vi "PXI-4130 Channel Section Page.vi"(8 "error in (no error)":errorcluster, 11 "Node Ptr":T3 format="%.0x") -> (0 "error out":errorcluster)   [LabVIEW 2009, in "PXI-4130 Custom Device.lvlib"]
uses:
  PXI-4130 Custom Device.lvlib
  <vilib>/NI VeriStand/Custom Device API/Custom Device Item Ref.ctl
  Channel Sense.ctl
  Channel Type.ctl
  <vilib>/NI VeriStand/Custom Device API/Get Item Property (I32).vi
  PXI-4130 Global Variable.vi
  <vilib>/NI VeriStand/Custom Device API/Set Item Property (I32).vi
  <vilib>/NI VeriStand/Custom Device API/Custom Device API.lvlib
panel:
  in  "Apply Change":bool
  in  "Channel Type":T1 caption="Channel 0 Sense" items=["Voltage Controlled", "Current Controlled"]
  in  "Channel Sense":T2=1008 caption="Channel 0 Sense" items=["Local"=1008, "Remote"=1009]
  in  "Header":cluster{"Section Name":string}={"Section Name"="Custom Device Item Settings"}
  in  "Description":string
  in  "Name":string
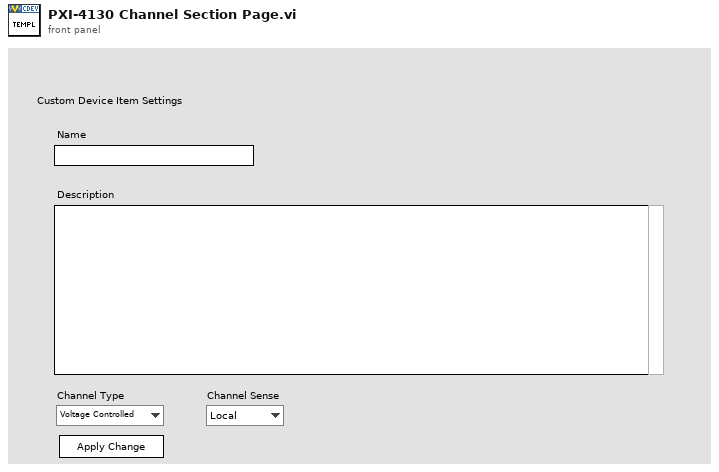
[diagram p1: front panel]
types:
  T1 = typedef "PXI-4130 Custom Device.lvlib/Channel Type.ctl" = i32
  T2 = typedef "PXI-4130 Custom Device.lvlib/Channel Sense.ctl" = i32
  T3 = typedef "Custom Device API.lvlib/Custom Device Item Ref.ctl" = u64
  T4 = enum8{"Enabled", "Disabled", "Disabled and Grayed Out"}
  T5 = typedef "Custom Device API.lvlib/Custom Device Item Info.ctl" = cluster{"Name":string, "Is Channel":bool, "GUID":string}
  T6 = typedef "Custom Device API.lvlib/Custom Device Commands.ctl" = enum16{"Default", "Item renamed", "Shutdown"}
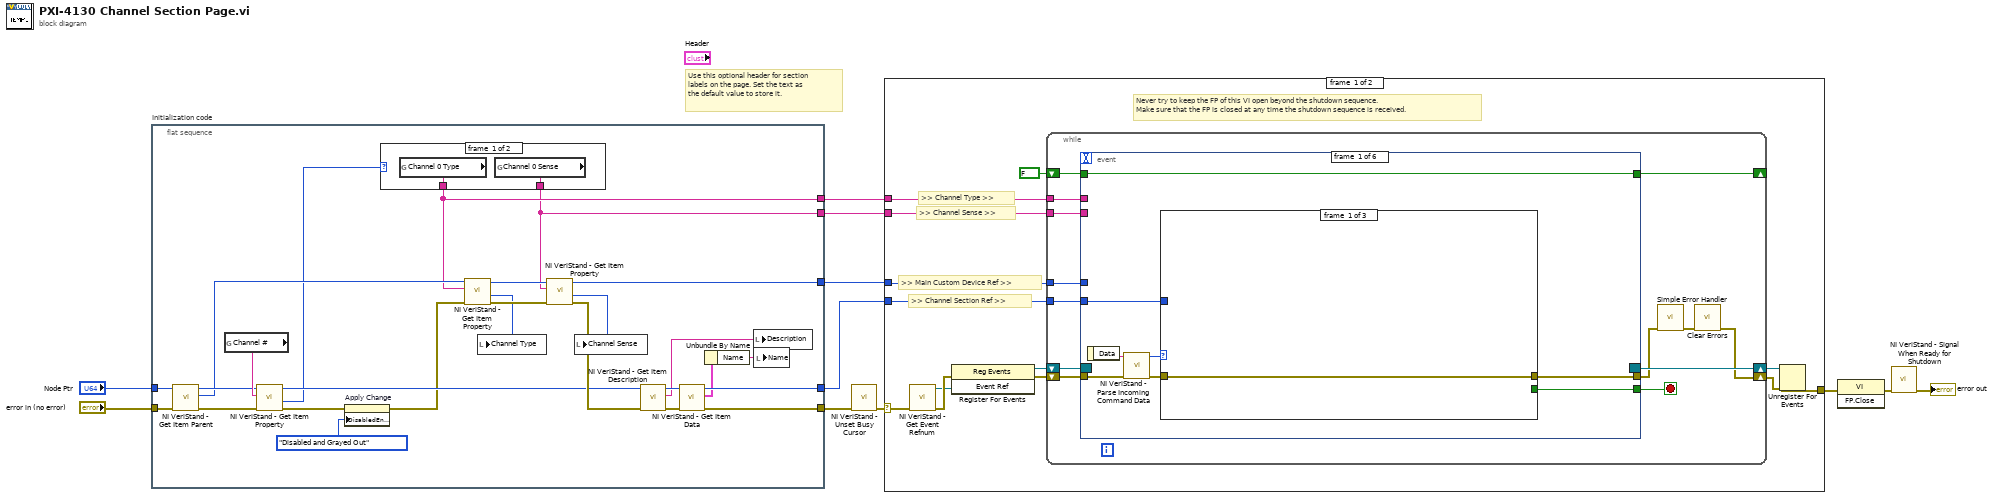
[diagram p0: block diagram]
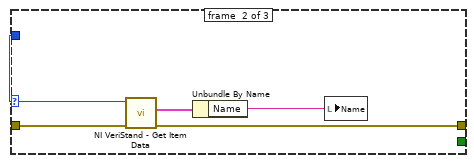
[diagram p2: hidden frame]
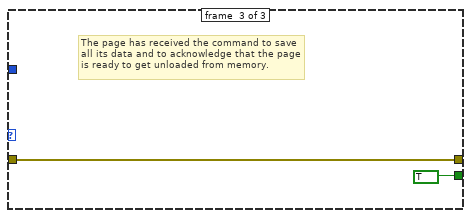
[diagram p3: hidden frame]
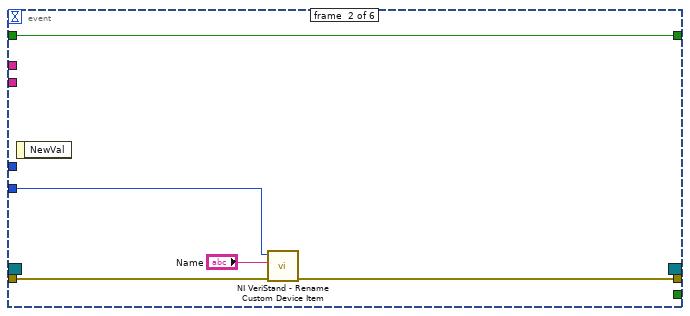
[diagram p4: hidden frame]
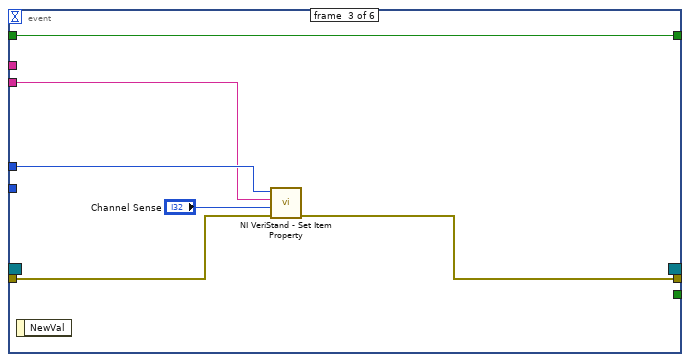
[diagram p5: hidden frame]
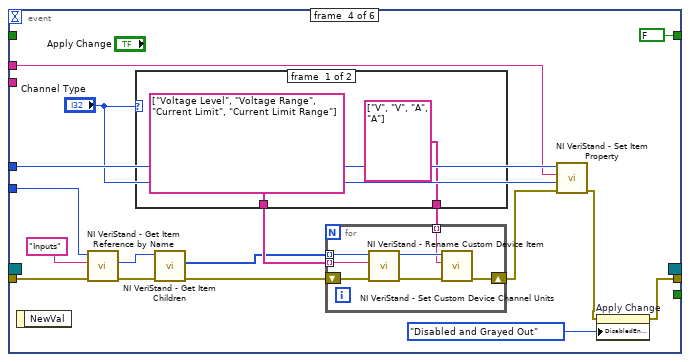
[diagram p6: hidden frame]
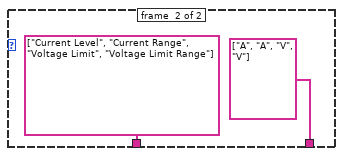
[diagram p7: hidden frame]
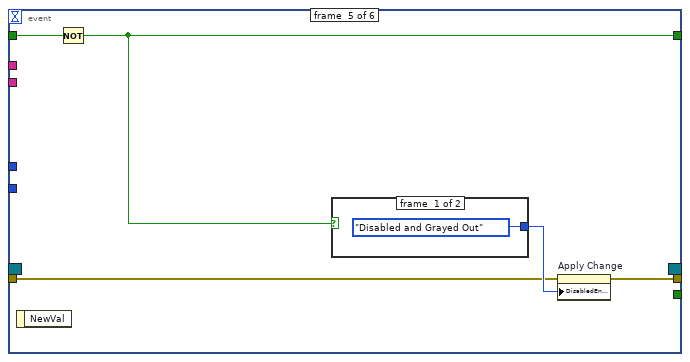
[diagram p8: hidden frame]
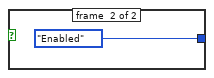
[diagram p9: hidden frame]
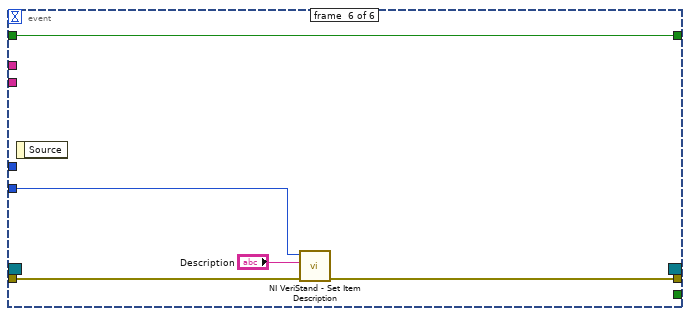
[diagram p10: hidden frame]
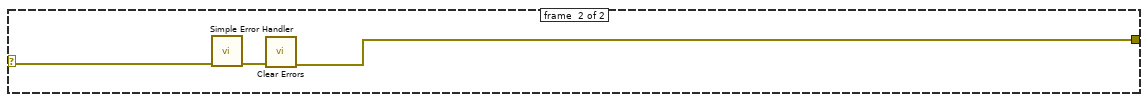
[diagram p11: hidden frame]
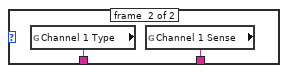
[diagram p12: hidden frame]
diagram:
  # "Use this optional header for section labels on the page. Set the text as the default value to store it."
  n1 = flat-sequence "Initialization code" {
    tunnel: "error in (no error)" -> [w28]
    tunnel: "Node Ptr" -> [w29]
    tunnel: [w31] -> w7
    tunnel: [w37] -> w4
    tunnel: [w18] -> w3
    tunnel: [w12] -> w2
    tunnel: [w13] -> w1
    frame #0 {
      n2 = call <vilib>:"NI VeriStand - Get Item Parent.vi"("error in (no error)"=w28, "Parent Ref in"=w29) -> ("error out"=w26:errorcluster, "Parent Ref"=w19:T3, "Parent Ref out"=w27:T3)  [unwired: 6 in, 1 out]
      n3 = global read "PXI-4130 Global Variable.vi" "Channel #"() -> (w30:string)
      n4 = call-poly <vilib>:"NI VeriStand - Get Item Property.vi"("error in (no error)"=w26, "Property Name"=w30, "Item Ref in"=w27) -> ("error out"=w16:errorcluster, "Value"=w14:i32, "Item Ref out"=w20:T3)  [unwired: 5 in, 1 out]
      n5 = property on="Apply Change" class="Bool"(error in=w16, "DisabledEnum"=T4."Disabled and Grayed Out" ("Disabled")) -> (error out=w15:errorcluster)  [unwired: 1 in, 1 out]
      n6 = case shown="0, Default" w14 {
        tunnel: [w39 w41] -> w13
        tunnel: [w38 w40] -> w12
        frame #0 {
          n7 = global read "PXI-4130 Global Variable.vi" "Channel 0 Type"() -> (w39:string)
          n8 = global read "PXI-4130 Global Variable.vi" "Channel 0 Sense"() -> (w38:string)
        }
        frame #1 {
          n9 = global read "PXI-4130 Global Variable.vi" "Channel 1 Type"() -> (w41:string)
          n10 = global read "PXI-4130 Global Variable.vi" "Channel 1 Sense"() -> (w40:string)
        }
      }
      n11 = call-poly <vilib>:"NI VeriStand - Get Item Property.vi"("error in (no error)"=w15, "Property Name"=w13, "Item Ref in"=w19) -> ("error out"=w24:errorcluster, "Value"=w22:i32, "Item Ref out"=w25:T3)  [unwired: 5 in, 1 out]
      n12 = local write "Channel Type"(w22) -> ()
      n13 = call-poly <vilib>:"NI VeriStand - Get Item Property.vi"("error in (no error)"=w24, "Property Name"=w12, "Item Ref in"=w25) -> ("error out"=w23:errorcluster, "Value"=w21:i32, "Item Ref out"=w18:T3)  [unwired: 5 in, 1 out]
      n14 = local write "Channel Sense"(w21) -> ()
      n15 = call <vilib>:"NI VeriStand - Get Item Description.vi"("error in (no error)"=w23, "Item Ref in"=w20) -> ("error out"=w34:errorcluster, "Description"=w35:string, "Item Ref out"=w36:T3)  [unwired: 7 out]
      n16 = call <vilib>:"NI VeriStand - Get Item Data.vi"("error in (no error)"=w34, "Item Ref in"=w36) -> ("error out"=w31:errorcluster, "Item Info"=w33:T5, "Item Ref out"=w37:T3)  [unwired: 7 out]
      n17 = Unbundle By Name(w33) -> ("Name"=w32:string)
      n18 = local write "Description"(w35) -> ()
      n19 = local write "Name"(w32) -> ()
    }
  }
  n20 = call <vilib>:"NI VeriStand - Unset Busy Cursor.vi"("error in (no error)"=w7) -> ("error out"=w6:errorcluster)  [unwired: 10 out]
  n21 = case shown="No Error" w6 {
    selector: w6 -> [w46 w137]
    tunnel: [w51 w135] -> w11
    tunnel: w4 -> [w47 _]
    tunnel: w3 -> [w45 _]
    tunnel: w2 -> [w44 _]
    tunnel: w1 -> [w43 _]
    frame #0 {
      # ">> Channel Type >>"
      # ">> Channel Sense >>"
      # ">> Main Custom Device Ref >>"
      # ">> Channel Section Ref >>"
      # "Never try to keep the FP of this VI open beyond the shutdown sequence.\nMake sure that the FP is closed at any time the shutdown sequence is received."
      n22 = call <vilib>:"NI VeriStand - Get Event Refnum.vi"("error in (no error)"=w46) -> ("error out"=w54:errorcluster, "Event Ref"=w50:refnum<user-event>)  [unwired: 9 out]
      n23 = register-events(error in=w54, w50) -> (reference out=w48:refnum<event-registration>, error out=w49:errorcluster)  [unwired: 1 in]
      n24 = while {
        tunnel: w47 -> [w63]
        shift-right: [w60] -> w52
        shift-left: w49 -> [w66]
        shift-right: [w67] -> w53
        shift-left: w48 -> [w65]
        tunnel: w45 -> [w59]
        tunnel: w44 -> [w58]
        tunnel: w43 -> [w57]
        shift-right: [w55] -> _
        shift-left: FALSE -> [w56]
        stop <- w64 stop-if-true
        n25 = event shown="[3] \"Apply Change\": Value Change" {
          selector: w65 -> [_ _ _ _ _ _]
          dyn-events: [_ _ _ _ _ _] -> w67
          timeout: _ -> [_ _ _ _ _ _]
          tunnel: w66 -> [w75 w88 w94 w108 w126 w133]
          tunnel: [w71 _ _ _ _ _] -> w64
          tunnel: [w70 w87 w93 w96 w125 w132] -> w62
          tunnel: w63 -> [w69 w86 _ w111 _ w134]
          tunnel: w59 -> [_ _ w91 w102 _ _]
          tunnel: w58 -> [_ _ w90 _ _ _]
          tunnel: w57 -> [_ _ _ w101 _ _]
          tunnel: w56 -> [w68 w84 w89 _ w124 w130]
          tunnel: [w68 w84 w89 FALSE w123 w130] -> w55
          event #0 {
            n26 = event-data() -> ("Data"=w74:string)  [unwired: 1 out]
            n27 = call <vilib>:"NI VeriStand - Parse Incoming Command Data.vi"("error in (no error)"=w75, "Data"=w74) -> ("error out"=w73:errorcluster, "Action"=w72:T6)  [unwired: 8 out]
            n28 = case shown="\"Shutdown\"" w72 {
              tunnel: w73 -> [w76 w81 w82]
              tunnel: [_ _ TRUE] -> w71
              tunnel: [w76 w78 w82] -> w70
              tunnel: w69 -> [_ w80 _]
              frame #0 {
              }
              frame #1 {
                n29 = call <vilib>:"NI VeriStand - Get Item Data.vi"("error in (no error)"=w81, "Item Ref in"=w80) -> ("error out"=w78:errorcluster, "Item Info"=w79:T5)  [unwired: 8 out]
                n30 = Unbundle By Name(w79) -> ("Name"=w77:string)
                n31 = local write "Name"(w77) -> ()
              }
              frame #2 {
                # "The page has received the command to save all its data and to acknowledge that the page is ready to get unloaded from memory."
              }
            }
          }
          event #1 {
            n32 = event-data() -> ()  [unwired: 2 out]
            n33 = call <vilib>:"NI VeriStand - Rename Custom Device Item.vi"("error in (no error)"=w88, "New Name"="Name", "Item Ref in"=w86) -> ("error out"=w87:errorcluster)  [unwired: 8 out]
          }
          event #2 {
            n34 = event-data() -> ()  [unwired: 2 out]
            n35 = call-poly <vilib>:"NI VeriStand - Set Item Property.vi"("error in (no error)"=w94, "Value"="Channel Sense", "Property Name"=w90, "Item Ref in"=w91) -> ("error out"=w93:errorcluster)  [unwired: 5 in, 2 out]
          }
          event #3 {
            n36 = event-data() -> ()  [unwired: 2 out]
            n37 = call <vilib>:"NI VeriStand - Get Item Reference by Name.vi"("error in (no error)"=w108, "Item Name"="Inputs", "Parent Ref in"=w111) -> ("error out"=w109:errorcluster, "Item Ref"=w105:T3)  [unwired: 5 in, 2 out]
            n38 = case shown="1" "Channel Type" {
              tunnel: [string[] ["Voltage Level", "Voltage Range", "Current Limit", "Current Limit Range"] string[] ["Current Level", "Current Range", "Voltage Limit", "Voltage Limit Range"]] -> w107
              tunnel: [string[] ["V", "V", "A", "A"] string[] ["A", "A", "V", "V"]] -> w99
              frame #0 {
              }
              frame #1 {
              }
            }
            n39 = call <vilib>:"NI VeriStand - Get Item Children.vi"("error in (no error)"=w109, "Item Ref in"=w105) -> ("error out"=w106:errorcluster, "Child Refs"=w104:T3[])  [unwired: 6 in, 2 out]
            n40 = for {
              tunnel: w107 -> [w118] mode=indexing
              tunnel: w104 -> [w117] mode=indexing
              shift-right: [w114] -> w103
              shift-left: w106 -> [w116]
              tunnel: w99 -> [w112] mode=indexing
              n41 = call <vilib>:"NI VeriStand - Rename Custom Device Item.vi"("error in (no error)"=w116, "New Name"=w118, "Item Ref in"=w117) -> ("error out"=w115:errorcluster, "Item Ref out"=w113:T3)  [unwired: 6 in, 1 out]
              n42 = call <vilib>:"NI VeriStand - Set Custom Device Channel Units.vi"("error in (no error)"=w115, "Units"=w112, "Channel Ref in"=w113) -> ("error out"=w114:errorcluster)  [unwired: 7 in, 1 out]
            }
            n43 = call-poly <vilib>:"NI VeriStand - Set Item Property.vi"("error in (no error)"=w103, "Value"="Channel Type", "Property Name"=w101, "Item Ref in"=w102) -> ("error out"=w97:errorcluster)  [unwired: 5 in, 2 out]
            n44 = property on="Apply Change" class="Bool"(error in=w97, "DisabledEnum"=T4."Disabled and Grayed Out" ("Disabled")) -> (error out=w96:errorcluster)  [unwired: 1 in, 1 out]
          }
          event #4 {
            n45 = event-data() -> ()  [unwired: 2 out]
            n46 = Not(x=w124) -> (.not. x?=w123:bool)
            n47 = case shown="True" w123 {
              tunnel: [T4."Disabled and Grayed Out" ("Disabled") T4."Enabled" ("Disabled")] -> w127
              frame #0 {
              }
              frame #1 {
              }
            }
            n48 = property on="Apply Change" class="Bool"(error in=w126, "DisabledEnum"=w127) -> (error out=w125:errorcluster)  [unwired: 1 in, 1 out]
          }
          event #5 {
            n49 = event-data() -> ()  [unwired: 2 out]
            n50 = call <vilib>:"NI VeriStand - Set Item Description.vi"("error in (no error)"=w133, "Description"="Description", "Item Ref in"=w134) -> ("error out"=w132:errorcluster)  [unwired: 8 out]
          }
        }
        n51 = call <vilib>:"Simple Error Handler.vi"("error in (no error)"=w62) -> ("error out"=w61:errorcluster)  [unwired: 1 in, 7 out]
        n52 = call <vilib>:"Clear Errors.vi"("error in (no error)"=w61) -> ("error out"=w60:errorcluster)  [unwired: 6 out]
      }
      n53 = Unregister For Events(event registration refnum=w53, error in=w52) -> (error out=w51:errorcluster)
    }
    frame #1 {
      n54 = call <vilib>:"Simple Error Handler.vi"("error in (no error)"=w137) -> ("error out"=w136:errorcluster)  [unwired: 1 in, 7 out]
      n55 = call <vilib>:"Clear Errors.vi"("error in (no error)"=w136) -> ("error out"=w135:errorcluster)  [unwired: 6 out]
    }
  }
  n56 = invoke class="VI" method="FP.Close"(error in=w11) -> (error out=w10:errorcluster)  [unwired: 2 in, 2 out]
  n57 = call <vilib>:"NI VeriStand - Signal When Ready for Shutdown.vi"("error in (no error)"=w10) -> ("error out"=→"error out":errorcluster)  [unwired: 10 out]
